vi "Generate Colour Table.vi"(1 "Code 320 Values":u16[](array[numeric])) -> (0 "Colour Table":u32[](array[colorbox]))   [LabVIEW 2013, in "Tiff reader.lvlib"]
doc: "Converts a colour table as specified in the tiff format into an array of labview colours."
uses:
  Tiff reader.lvlib
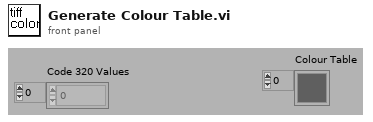
[diagram p1: front panel]
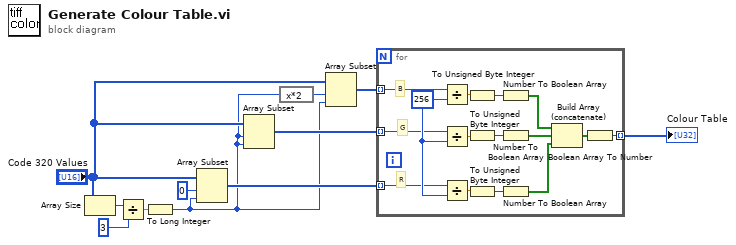
[diagram p0: block diagram]
diagram:
  n1 = Array Size(array="Code 320 Values") -> (size(s)=w11:i32)
  n2 = Divide(x=w11, y=3) -> (x/y=w2:dbl)
  n3 = To Long Integer(number=w2) -> (32bit integer=w1:i32)
  n4 = Array Subset(array="Code 320 Values", index=0 ("Array Index"), length=w1) -> (w7:u16[])
  n5 = Array Subset(array="Code 320 Values", index=w1, length=w1) -> (w6:u16[])
  n6 = expression code="x*2"(w1) -> (w3:i32)
  n7 = Array Subset(array="Code 320 Values", index=w3, length=w1) -> (w4:u16[])
  n8 = for {
    tunnel: [w17] -> w9 mode=indexing
    tunnel: w7 -> [w16] mode=indexing
    tunnel: w6 -> [w15] mode=indexing
    tunnel: w4 -> [w14] mode=indexing
    w26 = u16 256 ("y")
    # "B"
    # "G"
    # "R"
    n9 = Divide(x=w14, y=w26) -> (x/y=w25:dbl)
    n10 = Divide(x=w15, y=w26) -> (x/y=w24:dbl)
    n11 = Divide(x=w16, y=w26) -> (x/y=w23:dbl)
    n12 = To Unsigned Byte Integer(number=w25) -> (unsigned 8bit integer=w22:u8)
    n13 = To Unsigned Byte Integer(number=w24) -> (unsigned 8bit integer=w21:u8)
    n14 = To Unsigned Byte Integer(number=w23) -> (unsigned 8bit integer=w20:u8)
    n15 = Number To Boolean Array(number=w22) -> (Boolean array=w12:bool[])
    n16 = Number To Boolean Array(number=w21) -> (Boolean array=w19:bool[])
    n17 = Number To Boolean Array(number=w20) -> (Boolean array=w13:bool[])
    n18 = Build Array (concatenate)(w12, w19, w13) -> (w18:bool[])
    n19 = Boolean Array To Number(Boolean array=w18) -> (number=w17:u32)
  }
  "Colour Table" <- w9
